vi "Drive.GetSpeedDem.vi"() -> (2 "RSpeedDemand (ft/s)":dbl, 3 "LSpeedDemand (ft/s)":dbl)   [LabVIEW 2020]
doc: "Get speed demand variable for drive"
uses:
  Drive.Global.vi
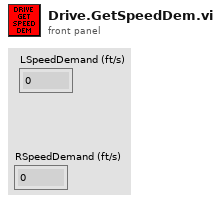
[diagram p1: front panel]
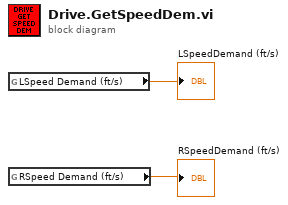
[diagram p0: block diagram]
diagram:
  n1 = global read "Drive.Global.vi" "LSpeed Demand (ft/s)"() -> (→"LSpeedDemand (ft/s)":dbl)
  n2 = global read "Drive.Global.vi" "RSpeed Demand (ft/s)"() -> (→"RSpeedDemand (ft/s)":dbl)
